vi "De-Initialize.vi"(8 "error in (no error)":errorcluster, 11 "DAQmx Digitizer in":refnum<class "DAQmx Synthesizer.lvclass">) -> (0 "error out":errorcluster, 3 "DAQmx Digitizer out":refnum<class "DAQmx Synthesizer.lvclass">)   [LabVIEW 2019, in "DAQmx Synthesizer.lvclass"]
uses:
  DAQmx Synthesizer.lvclass
  DAQmx Synthesizer.lvclass/DAQmx Synthesizer.ctl
  Instruments/Pulse Driver/Pulse Driver.lvclass
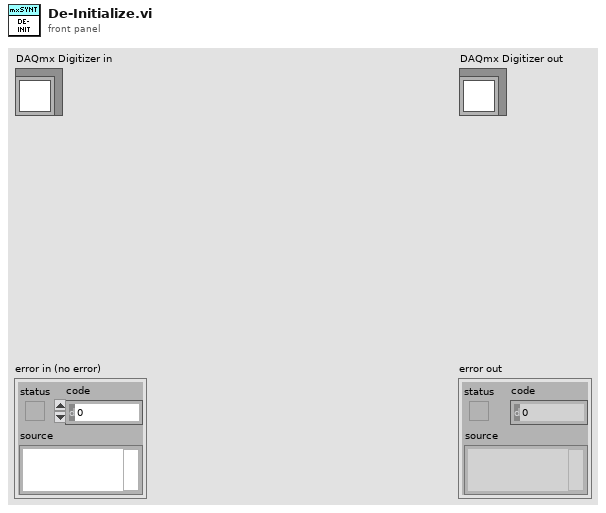
[diagram p1: front panel]
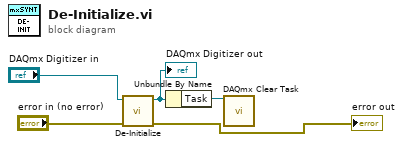
[diagram p0: block diagram]
diagram:
  n1 = call-parent "De-Initialize.vi"("error in (no error)"="error in (no error)", "Instrument Driver in"="DAQmx Digitizer in") -> ("error out"=→"error out":errorcluster, "Instrument Driver out"=w3:refnum<class "DAQmx Synthesizer.lvclass">)  [unwired: 8 in]
  "DAQmx Digitizer out" <- w3
  n2 = Unbundle By Name(w3) -> ("Task"=w1:refnum<k21>)
  n3 = call <vilib>:"DAQmx Clear Task.vi"("task in"=w1) -> ()  [unwired: 14 in, 1 out]
